vi "High G open csv.vi"(0 "file path":path, 11 "error in (no error)":errorcluster) -> (6 "X axis":dbl[](array[numeric]), 8 "Y axis":dbl[](array[numeric]), 10 "Z axis":dbl[](array[numeric]), 15 "error out":errorcluster)   [LabVIEW 2011]
uses:
  Stroker/High G/high G data GFV Action.ctl
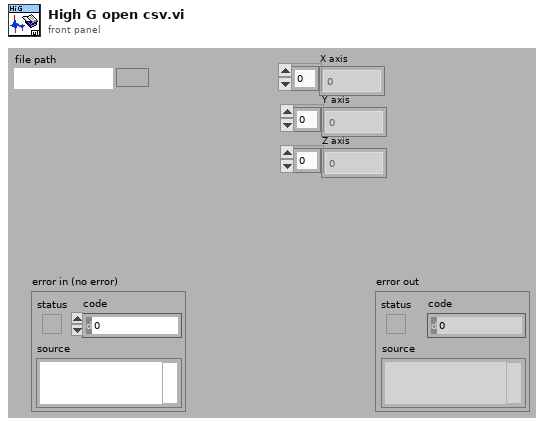
[diagram p1: front panel]
types:
  T1 = enum16{"open", "replace", "create", "open or create", "replace or create", "replace or create with confirmation"}
  T2 = typedef "high G data GFV Action.ctl" = enum16{"Init", "Add data", "Get"}
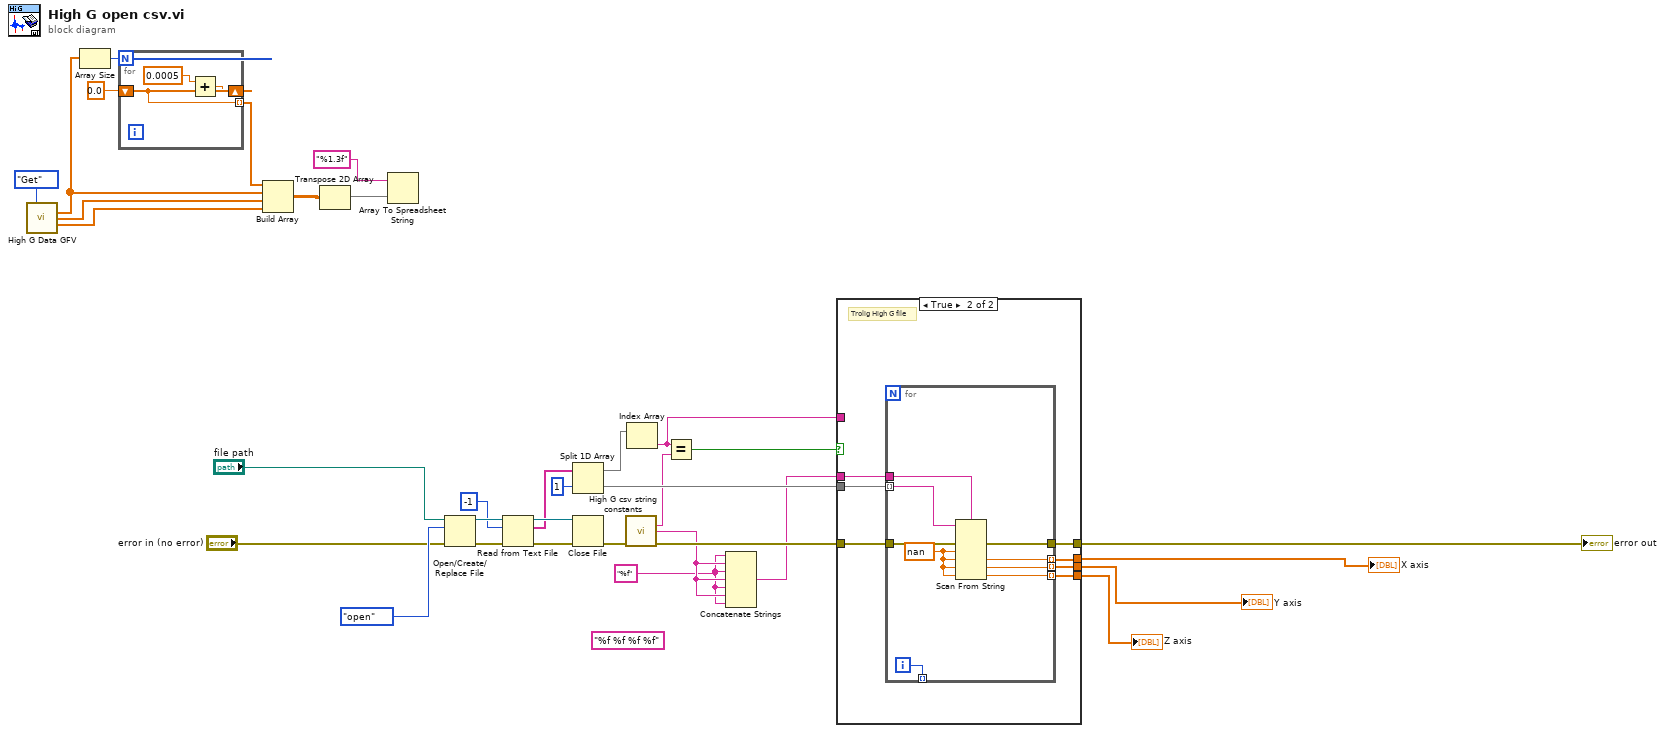
[diagram p0: block diagram]
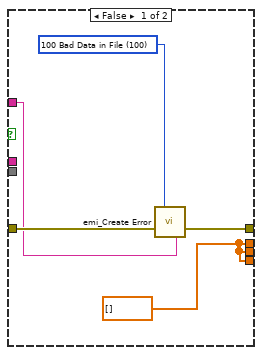
[diagram p2: hidden frame]
diagram:
  w1 = "%f"
  (unwired) "%f %f %f %f" ("format string")
  n1 = call "High G Data GFV.vi"("Action"=high_G_data_GFV_Action."Get") -> ("X axis"=w26:dbl[], "Y axis"=w25:dbl[], "Z axis"=w24:dbl[])  [unwired: 10 in, 2 out]
  n2 = Array Size(array=w26) -> (size(s)=w29:i32)
  n3 = for {
    N: w29 -> [_]
    tunnel: [w37] -> w27 mode=indexing
    shift-right: [w36] -> _
    shift-left: 0.0 -> [w37]
    n4 = Add(x=0.0005, y=w37) -> (x+y=w36:dbl)
  }
  n5 = Build Array(w27, w26, w25, w24) -> (w30:dbl[][])
  n6 = Transpose 2D Array(2D array=w30) -> (transposed array=w32:dbl[][])
  n7 = Array To Spreadsheet String(array=w32, 3:"%1.3f" ("format string")) -> ()  [unwired: 1 in, 1 out]
  n8 = Open/Create/Replace File(file path (use dialog)="file path", error in="error in (no error)", operation (0:open)=T1."open") -> (refnum out=w20:refnum<file>, error out=w21:errorcluster)  [unwired: 3 in, 1 out]
  n9 = Read from Text File(file (use dialog)=w20, count=-1, error in=w21) -> (refnum out=w19:refnum<file>, text=w16:string[], error out=w17:errorcluster)  [unwired: 1 in, 1 out]
  n10 = Split 1D Array(array=w16, index=1) -> (first subarray=w12:string[], second subarray=w13:string[])
  n11 = Close File(refnum=w19, error in=w17) -> (error out=w15:errorcluster)  [unwired: 1 out]
  n12 = call "High G csv string constants.vi"("error in (no error)"=w15) -> ("Header"=w11:string, "Delimiter"=w2:string, "error out"=w9:errorcluster)  [unwired: 11 in, 1 out]
  n13 = Index Array(array=w12) -> (element=w3:string)  [unwired: 1 in]
  n14 = Equal?(x=w3, y=w11) -> (x = y?=w10:bool)
  n15 = Concatenate Strings(w1, w2, w1, w2, w1, w2, w1) -> (w8:string)
  n16 = case shown="True" w10 {
    tunnel: w13 -> [_ w49]
    tunnel: w9 -> [w41 w47]
    tunnel: w8 -> [_ w48]
    tunnel: [w40 w46] -> w7
    tunnel: [w42 w45] -> w6
    tunnel: [w42 w44] -> w5
    tunnel: [w42 w43] -> w4
    tunnel: w3 -> [w38 _]
    frame False {
      w39 = 100 items=["0 No Error"=0, "1 Invalid input parameter"=1, "6 Generic file IO "=6, "7 File not Found"=7, "35 Generic Pring Error"=35, "37 Device not Found"=37, "39 Device Unit Error"=39, "40 Could fot Open Device"=40, "42 Generic Error"=42, "52 Unknown Message"=52, "98 Bad File type"=98, "99 Bad File Version"=99, "100 Bad Data in File"=100, "1018 Unspecefied Error"=1018, "1041 Incorrect Password"=1041, "1043 Feature not in this version"=1043, "1109 Unsuported Data type"=1109, "1444 Did not close sucessfully"=1444] ("Error Code")
      w42 = dbl[] []
      n17 = call "emi_Create Error.vi"("Error Code"=w39, "error in (no error)"=w41, "Append String(\"\")"=w38) -> ("error out"=w40:errorcluster)  [unwired: 12 in]
    }
    frame True {
      # "Trolig High G file"
      n18 = for {
        tunnel: w49 -> [w58] mode=indexing
        tunnel: w48 -> [w57]
        tunnel: w47 -> [w56]
        tunnel: [w54] -> w45 mode=indexing
        tunnel: [w53] -> w44 mode=indexing
        tunnel: [w52] -> w43 mode=indexing
        tunnel: [w51] -> w46
        tunnel: [w50] -> _ mode=indexing
        i -> [w50]
        w55 = nan ("default value 1")
        n19 = Scan From String(format string=w57, input string=w58, error in=w56, default 1=w55, default 2=w55, default 3=w55, default 4=w55) -> (error out=w51:errorcluster, output 2=w54:dbl, output 3=w53:dbl, output 4=w52:dbl)  [unwired: 2 in, 2 out]
      }
    }
  }
  "error out" <- w7
  "X axis" <- w6
  "Y axis" <- w5
  "Z axis" <- w4
